vi "AdjustScalesIntervalSingle.vi"(7 "Action":enum16{"Init", "Set Scale"}(ring), 10 "WFChart Refnum":refnum<vi>) -> ()   [LabVIEW 2013, in "main.lvlib"]
uses:
  main.lvlib
  <vilib>/Utility/miscctls.llb/LVRangeTypeDef.ctl
  <vilib>/Analysis/baseanly.llb/Mean (DBL).vi
  <vilib>/Analysis/NI_AALBase.lvlib
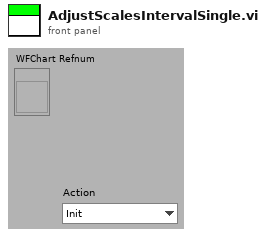
[diagram p1: front panel]
types:
  T1 = typedef "LVRangeTypeDef.ctl" = cluster{"Minimum":dbl, "Maximum":dbl, "Increment":dbl, "Minor Increment":dbl, "Start":dbl}
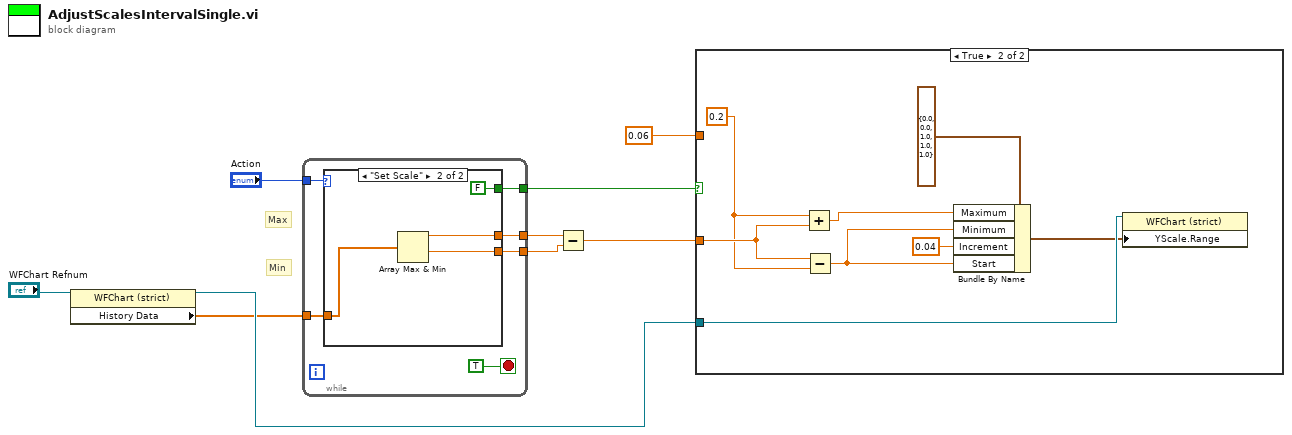
[diagram p0: block diagram]
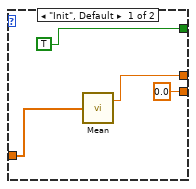
[diagram p2: hidden frame]
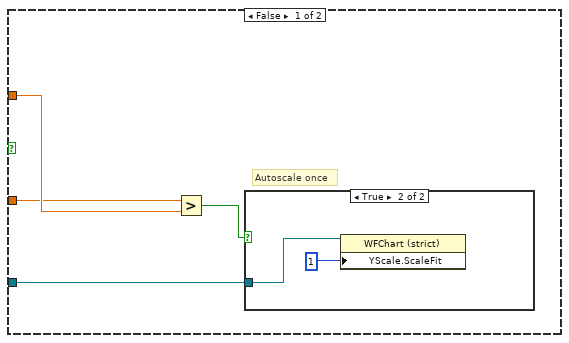
[diagram p3: hidden frame]
diagram:
  # "Min"
  # "Max"
  n1 = property class="WFChart (strict)"(reference="WFChart Refnum") -> ("History Data"=w4:dbl[])  [unwired: 1 in, 2 out]
  n2 = while {
    tunnel: "Action" -> [w13]
    tunnel: [w12] -> w7
    tunnel: w4 -> [w11]
    tunnel: [w10] -> w3
    tunnel: [w9] -> w2
    stop <- TRUE stop-if-true
    n3 = case shown="\"Set Scale\"" w13 {
      tunnel: w11 -> [w17 w21]
      tunnel: [TRUE FALSE] -> w12
      tunnel: [w16 w20] -> w10
      tunnel: [0.0 w19] -> w9
      frame "Init", Default {
        n4 = call-poly <vilib>:"Mean.vi"("X"=w17) -> ("mean"=w16:dbl)  [unwired: 1 out]
      }
      frame "Set Scale" {
        n5 = Array Max & Min(array=w21) -> (max value=w20:dbl, min value=w19:dbl)  [unwired: 2 out]
      }
    }
  }
  n6 = Subtract(x=w3, y=w2) -> (x-y=w1:dbl)
  n7 = case shown="True" w7 {
    tunnel: "WFChart Refnum" -> [w26 w36]
    tunnel: 0.06 ("x") -> [w24 _]
    tunnel: w1 -> [w23 w30]
    frame False {
      # "Autoscale once"
      n8 = Greater?(x=w23, y=w24) -> (0:w25:bool)
      n9 = case shown="True" w25 {
        tunnel: w26 -> [_ w28]
        frame False {
        }
        frame True {
          n10 = property class="WFChart (strict)"(reference=w28, "YScale.ScaleFit"=u8 1 ("Y Scale.Scale Fit")) -> ()  [unwired: 1 in, 2 out]
        }
      }
    }
    frame True {
      w29 = 0.2 ("x")
      n11 = Add(x=w29, y=w30) -> (x+y=w32:dbl)
      n12 = Subtract(x=w30, y=w29) -> (x-y=w33:dbl)
      n13 = Bundle By Name(cluster=T1 {"Minimum"=0.0, "Maximum"=0.0, "Increment"=1.0, "Minor Increment"=1.0, "Start"=1.0} ("Y Scale.Range"), "Maximum"=w32, "Minimum"=w33, "Increment"=0.04, "Start"=w33) -> (w31:T1)
      n14 = property class="WFChart (strict)"(reference=w36, "YScale.Range"=w31) -> ()  [unwired: 1 in, 2 out]
    }
  }
